vi "sTimer.vi"(8 "Time interval in":u64, 9 "Arduino read rate (Hz)":dbl=1.0, 10 "Updated NIST Time":u64, 11 "NIST Time In":u64) -> (0 "Time interval out":u64, 3 "NIST Time Out":u64)   [LabVIEW 2012]
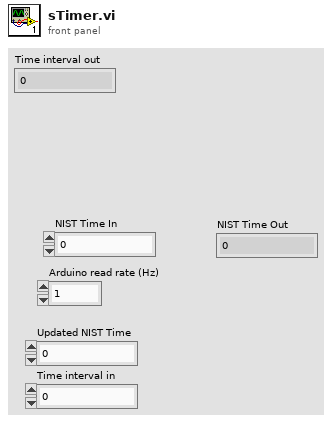
[diagram p1: front panel]
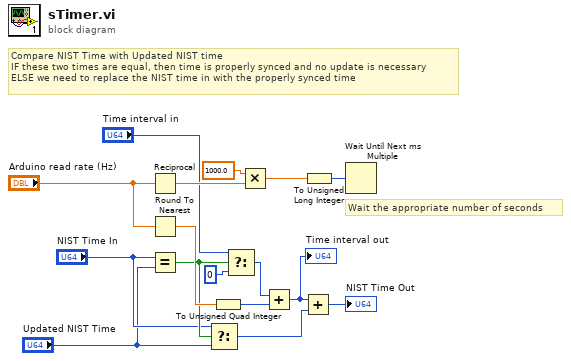
[diagram p0: block diagram]
diagram:
  # "Compare NIST Time with Updated NIST time\nIF these two times are equal, then time is properly synced and no update is necessary\nELSE we need to replace the NIST time in with the properly synced time"
  # "Wait the appropriate number of seconds"
  n1 = Reciprocal(x="Arduino read rate (Hz)") -> (1/x=w13:dbl)
  n2 = Round To Nearest(number="Arduino read rate (Hz)") -> (nearest integer value=w12:dbl)
  n3 = Equal?(x="NIST Time In", y="Updated NIST Time") -> (x = y?=w10:bool)
  n4 = Select(t="NIST Time In", s=w10, f="Updated NIST Time") -> (s? t:f=w2:u64)
  n5 = To Unsigned Quad Integer(1:w12) -> (0:w9:u64)
  n6 = Select(t="Time interval in", s=w10, f=u64 0) -> (s? t:f=w6:u64)
  n7 = Multiply(x=1000.0 ("millisecond multiple"), y=w13) -> (x*y=w15:dbl)
  n8 = Add(x=w6, y=w9) -> (x+y=w3:u64)
  "Time interval out" <- w3
  n9 = Add(x=w3, y=w2) -> (x+y=→"NIST Time Out":u64)
  n10 = To Unsigned Long Integer(number=w15) -> (unsigned 32bit integer=w14:u32)
  n11 = Wait Until Next ms Multiple(millisecond multiple=w14) -> ()  [unwired: 1 out]
